vi "Extract Tokens in Range.vi"(10 "tokens":cluster{"token type":T4, "info":T2}[](array[cluster]), 11 "range info":T1[](array[typedef])) -> (3 "tokens out":cluster{"token type":T4, "info":T2}[](array[cluster]))   [LabVIEW 2020, in "Multi Error Cluster.lvlib"]
doc: "Given tokens and desciptors for an element or object, return the subset of tokens."
uses:
  <vilib>/MultiError/TokenizeJSON/Multi Error Cluster.lvlib
  <vilib>/MultiError/TokenizeJSON/JSON Token Values.ctl
  <vilib>/MultiError/Errors Cluster Multiple Errors/JSON Token Descriptor.ctl
  <vilib>/MultiError/TokenizeJSON/JSON Raw Token Values.ctl
  <vilib>/MultiError/Errors Cluster Multiple Errors/JSON Object Descriptor.ctl
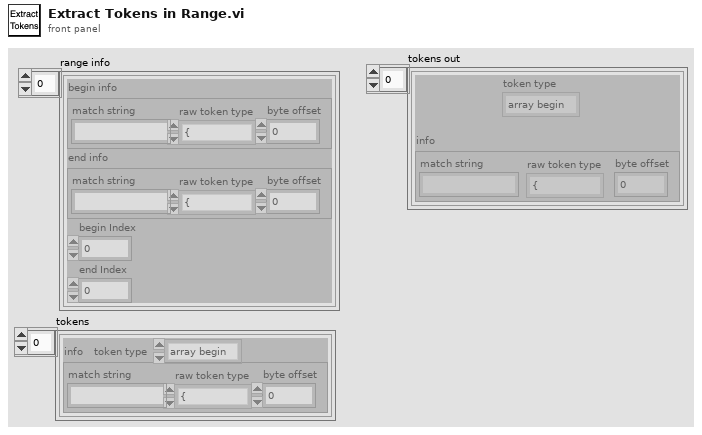
[diagram p1: front panel]
types:
  T1 = typedef "Multi Error Cluster.lvlib/JSON Object Descriptor.ctl" = cluster{"begin info":T2, "end info":T2, "begin Index":i32, "end Index":i32}
  T2 = typedef "Multi Error Cluster.lvlib/JSON Token Descriptor.ctl" = cluster{"match string":string, "raw token type":T3, "byte offset ":i32}
  T3 = typedef "Multi Error Cluster.lvlib/JSON Raw Token Values.ctl" = enum32{"{", "}", "[", "]", ",", ":", "\"", "number", "string", "true", "false", "null", "invalid"}
  T4 = typedef "Multi Error Cluster.lvlib/JSON Token Values.ctl" = enum32{"array begin", "array end", "object begin", "object end", "value", "invalid", "name"}
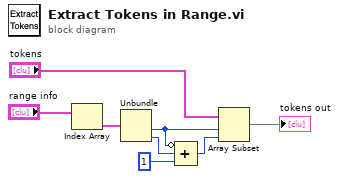
[diagram p0: block diagram]
diagram:
  n1 = Index Array(array="range info") -> (element=w2:T1)  [unwired: 1 in]
  n2 = Unbundle(w2) -> ("begin Index"=w6:i32, "end Index"=w4:i32)  [unwired: 2 out]
  n3 = Compound Arithmetic op=ADD(invert w6, w4, 1) -> (w5:i32)
  n4 = Array Subset(array="tokens", index=w6, length=w5) -> (→"tokens out":cluster{"token type":T4, "info":T2}[])
